vi "RPMEvent Read.vi"(4 "error in (no error)":errorcluster, 6 "Container State":T2, 7 "Display State In":T1) -> (0 "error out":errorcluster, 2 "Value":refnum<user-event>, 3 "Display State Out":T1)   [LabVIEW 2019, in "Gauge_pump.xctl"]
uses:
  Gauge_pump.xctl
  <vilib>/_xctls/Container State.ctl
  State _Gauge_pump.ctl
  <vilib>/_xctls/XControlSupport.lvlib
panel:
  # "Replace the Value Indicator below with an Indicator of desired type.\nDo not remove this Indicator or the others from the connector pane. \nDo not change the connector pane pattern.\nThe Value Indicator should always be the second terminal from top on the output side in the connector pane."
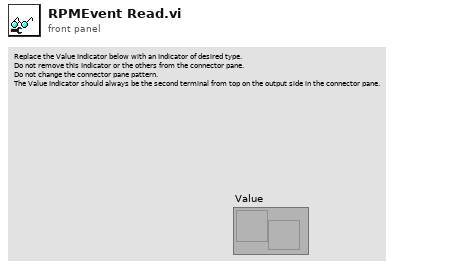
[diagram p1: front panel]
types:
  T1 = typedef "Gauge_pump.xctl/State _Gauge_pump.ctl" = cluster{"RPM":dbl, "direction":bool, "start/stop":bool, "RPMEvent":refnum<user-event>, "DirectionEvent":refnum<user-event>, "Start_stopEvent":refnum<user-event>}
  T2 = typedef "XControlSupport.lvlib/Container State.ctl" = cluster{"Indicator?":bool, "Run Mode?":bool, " Refnum":refnum<vi>}
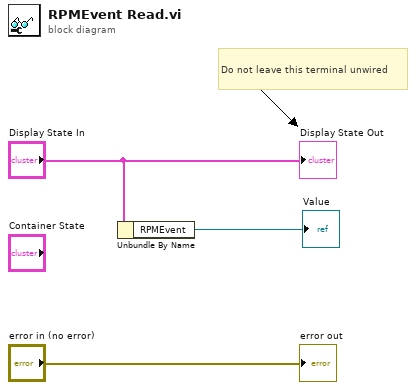
[diagram p0: block diagram]
diagram:
  # "Do not leave this terminal unwired"
  n1 = Unbundle By Name("Display State In") -> ("RPMEvent"=→"Value":refnum<user-event>)
  "error out" <- "error in (no error)"
  "Display State Out" <- "Display State In"
